vi "Create_VI_Doc_Component_Img_and_HTML.vi"(6 "special chars in file path of image":string, 7 "Content Options":T1, 8 "error in (no error)":errorcluster, 9 "Image Depth":i32=24, 10 "Image Format (jpeg)":enum32{"PNG", "JPEG", "GIF"}(ring)=enum."JPEG", 11 "VI":refnum<vi>) -> (0 "error out":errorcluster, 2 "HTML File Path":path, 3 "Path to image":path)   [LabVIEW 2020, in "NI_ReportGenerationCore.lvlib"]
uses:
  <vilib>/Utility/NIReport.llb/NI_ReportGenerationCore.lvlib
  <vilib>/printing/ReportDocExtensions.llb/File_types_for_reports.ctl
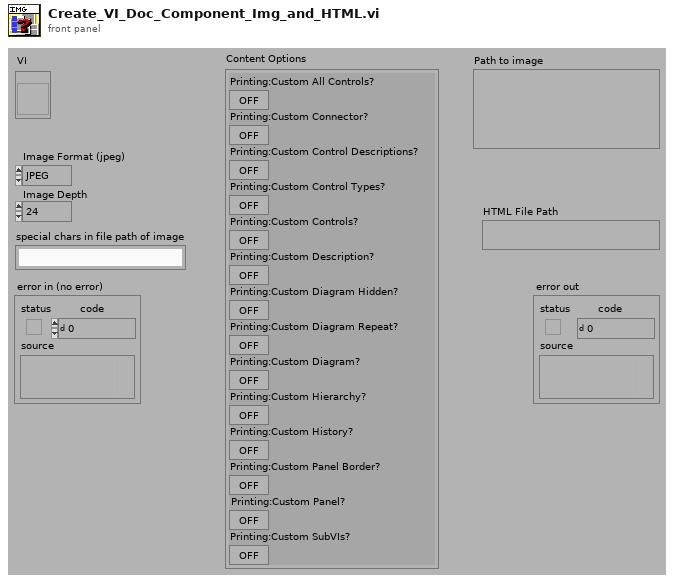
[diagram p1: front panel]
types:
  T1 = cluster{"Printing:Custom All Controls?":bool, "Printing:Custom Connector?":bool, "Printing:Custom Control Descriptions?":bool, "Printing:Custom Control Types?":bool, "Printing:Custom Controls?":bool, "Printing:Custom Description?":bool, "Printing:Custom Diagram Hidden?":bool, "Printing:Custom Diagram Repeat?":bool, "Printing:Custom Diagram?":bool, "Printing:Custom Hierarchy?":bool, "Printing:Custom History?":bool, "Printing:Custom Panel Border?":bool, "Printing:Custom Panel?":bool, "Printing:Custom SubVIs?":bool}
  T2 = typedef "NI_ReportGenerationCore.lvlib/File_types_for_reports.ctl" = enum16{".jpg", ".png", ".html", ".gif"}
  T3 = enum32{"Custom", "Standard", "Using Panel", "Using SubVI", "Complete"}
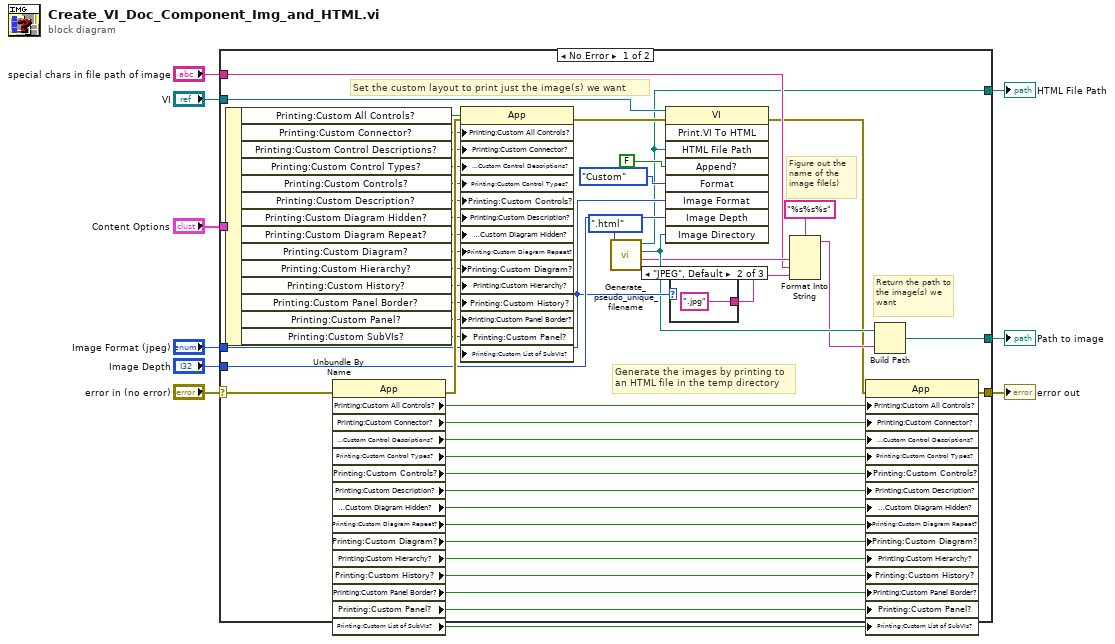
[diagram p0: block diagram]
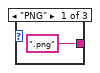
[diagram p2: hidden frame]
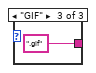
[diagram p3: hidden frame]
diagram:
  n1 = case shown="No Error" "error in (no error)" {
    selector: "error in (no error)" -> [w11 w61]
    tunnel: [w43 w61] -> w9
    tunnel: "VI" -> [w40 _]
    tunnel: "Image Depth" -> [w39 _]
    tunnel: [w10 _] -> w6
    tunnel: "Image Format (jpeg)" -> [w34 _]
    tunnel: [w31 _] -> w4
    tunnel: "Content Options" -> [w29 _]
    tunnel: "special chars in file path of image" -> [w13 _]
    frame No Error {
      # "Figure out the name of the image file(s)"
      # "Return the path to the image(s) we want"
      # "Generate the images by printing to an HTML file in the temp directory"
      # "Set the custom layout to print just the image(s) we want"
      n2 = Unbundle By Name(w29) -> ("Printing:Custom All Controls?"=w28:bool, "Printing:Custom Connector?"=w27:bool, "Printing:Custom Control Descriptions?"=w26:bool, "Printing:Custom Control Types?"=w25:bool, "Printing:Custom Controls?"=w24:bool, "Printing:Custom Description?"=w23:bool, "Printing:Custom Diagram Hidden?"=w22:bool, "Printing:Custom Diagram Repeat?"=w21:bool, "Printing:Custom Diagram?"=w20:bool, "Printing:Custom Hierarchy?"=w19:bool, "Printing:Custom History?"=w18:bool, "Printing:Custom Panel Border?"=w17:bool, "Printing:Custom Panel?"=w16:bool, "Printing:Custom SubVIs?"=w15:bool)
      n3 = property class="App"(error in=w11) -> (error out=w42:errorcluster, "Printing:Custom All Controls?"=w44:bool, "Printing:Custom Connector?"=w45:bool, "Printing:Custom Control Descriptions?"=w46:bool, "Printing:Custom Control Types?"=w47:bool, "Printing:Custom Controls?"=w48:bool, "Printing:Custom Description?"=w49:bool, "Printing:Custom Diagram Hidden?"=w50:bool, "Printing:Custom Diagram Repeat?"=w51:bool, "Printing:Custom Diagram?"=w52:bool, "Printing:Custom Hierarchy?"=w53:bool, "Printing:Custom History?"=w54:bool, "Printing:Custom Panel Border?"=w55:bool, "Printing:Custom Panel?"=w56:bool, "Printing:Custom List of SubVIs?"=w57:bool)  [unwired: 1 in, 1 out]
      n4 = property class="App"(error in=w42, "Printing:Custom All Controls?"=w28, "Printing:Custom Connector?"=w27, "Printing:Custom Control Descriptions?"=w26, "Printing:Custom Control Types?"=w25, "Printing:Custom Controls?"=w24, "Printing:Custom Description?"=w23, "Printing:Custom Diagram Hidden?"=w22, "Printing:Custom Diagram Repeat?"=w21, "Printing:Custom Diagram?"=w20, "Printing:Custom Hierarchy?"=w19, "Printing:Custom History?"=w18, "Printing:Custom Panel Border?"=w17, "Printing:Custom Panel?"=w16, "Printing:Custom List of SubVIs?"=w15) -> (error out=w41:errorcluster)  [unwired: 1 in, 1 out]
      n5 = call <vilib>:"Generate_pseudo_unique_filename.vi"("file type(.jpg)"=File_types_for_reports.".html") -> ("root filename"=w30:string, "temp directory"=w33:path, "generated path"=w10:path)  [unwired: 8 in]
      n6 = invoke class="VI" method="Print.VI To HTML"(reference=w40, error in=w41, "HTML File Path"=w10, "Append?"=FALSE, "Format"=T3."Custom", "Image Format"=w34, "Image Depth"=w39, "Image Directory"=w33) -> (error out=w12:errorcluster)  [unwired: 1 in, 8 out]
      n7 = case shown="\"JPEG\", Default" w34 {
        tunnel: [".png" ".jpg" ".gif"] -> w14
        frame "PNG" {
        }
        frame "JPEG", Default {
        }
        frame "GIF" {
        }
      }
      n8 = Format Into String(format string="%s%s%s" ("Format String"), w30, w13, w14) -> (resulting string=w32:string)  [unwired: 2 in, 1 out]
      n9 = property class="App"(error in=w12, "Printing:Custom All Controls?"=w44, "Printing:Custom Connector?"=w45, "Printing:Custom Control Descriptions?"=w46, "Printing:Custom Control Types?"=w47, "Printing:Custom Controls?"=w48, "Printing:Custom Description?"=w49, "Printing:Custom Diagram Hidden?"=w50, "Printing:Custom Diagram Repeat?"=w51, "Printing:Custom Diagram?"=w52, "Printing:Custom Hierarchy?"=w53, "Printing:Custom History?"=w54, "Printing:Custom Panel Border?"=w55, "Printing:Custom Panel?"=w56, "Printing:Custom List of SubVIs?"=w57) -> (error out=w43:errorcluster)  [unwired: 1 in, 1 out]
      n10 = Build Path(base path=w33, name or relative path=w32) -> (appended path=w31:path)
    }
    frame Error {
    }
  }
  "error out" <- w9
  "Path to image" <- w4
  "HTML File Path" <- w6
